vi "Eathquake n tsunami ver1.vi"() -> ()   [LabVIEW 2019]
panel:
  in  "Richter Scale":dbl(slide) scale=0.0..10.0
  out "Earthquake":bool
  out "Tsunami":bool
  out "Normal":bool
  out "x+y":i32
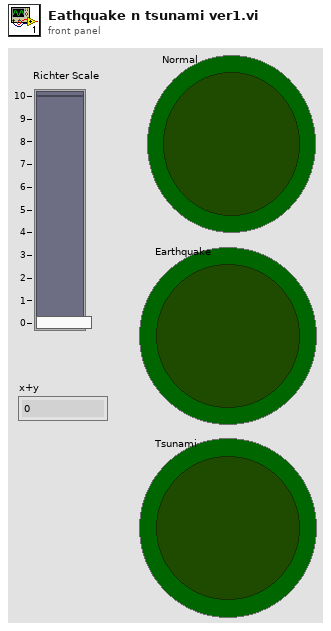
[diagram p1: front panel]
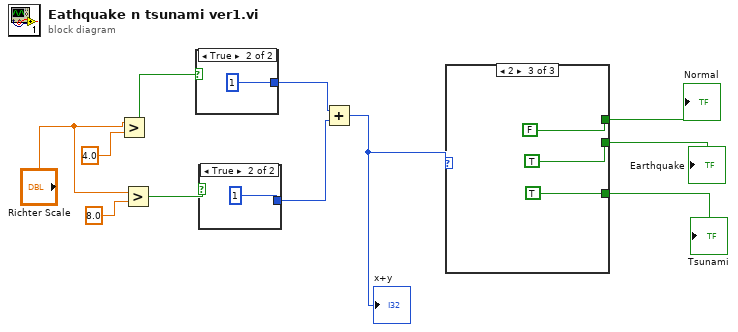
[diagram p0: block diagram]
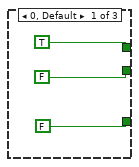
[diagram p2: hidden frame]
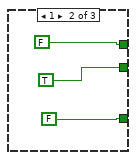
[diagram p3: hidden frame]
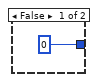
[diagram p4: hidden frame]
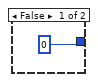
[diagram p5: hidden frame]
diagram:
  n1 = Greater?(x="Richter Scale", y=4.0) -> (0:w9:bool)
  n2 = Greater?(x="Richter Scale", y=8.0) -> (0:w8:bool)
  n3 = case shown="True" w9 {
    tunnel: [0 1] -> w7
    frame False {
    }
    frame True {
    }
  }
  n4 = case shown="True" w8 {
    tunnel: [0 1] -> w6
    frame False {
    }
    frame True {
    }
  }
  n5 = Add(x=w7, y=w6) -> (x+y=w5:i32)
  "x+y" <- w5
  n6 = case shown="2" w5 {
    tunnel: [TRUE FALSE FALSE] -> w4
    tunnel: [FALSE TRUE TRUE] -> w3
    tunnel: [FALSE FALSE TRUE] -> w2
    frame 0, Default {
    }
    frame 1 {
    }
    frame 2 {
    }
  }
  "Normal" <- w4
  "Tsunami" <- w2
  "Earthquake" <- w3
